vi "_SetTimeout.vi"(2 "tmo_in_msecs":u32, 3 "device_name":string) -> (0 "error stack":string[](array[string]), 1 "error code":i32)   [LabVIEW 2014, in "tango.lvlib"]
uses:
  tango.lvlib
  tango_binding.so
panel:
  # "This Vi is deprecated and only maintained for backward compatibility. Please use  _TangoSetTimeout instead."
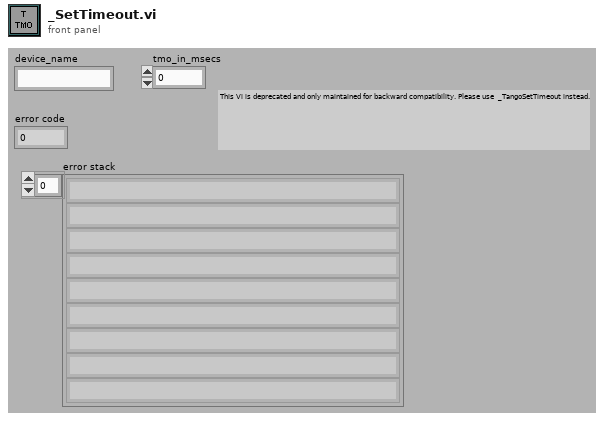
[diagram p1: front panel]
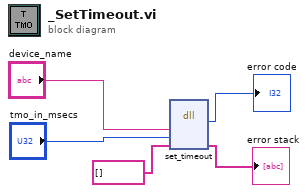
[diagram p0: block diagram]
diagram:
  n1 = dll-call lib="tango_binding.*" fn="set_timeout"("device_name"="device_name", "tmo_in_msecs"="tmo_in_msecs", "error_stack"=string[] [] ("error stack")) -> ("return type"=→"error code":i32, "error_stack"=→"error stack":string[])  [unwired: 5 in, 2 out]
